vi "DIO0 trigger.vi"(7 "Pulse ticks":u32=2, 8 "error in":errorcluster) -> (0 "error out":errorcluster)   [LabVIEW 2024]
uses:
  <vilib>/rvi/eio/common/nirviEmuTemplateMethod_errors.vi
  <vilib>/eio/EIONode/EIONode.xnode
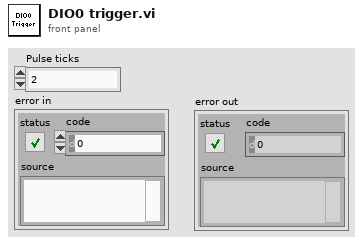
[diagram p1: front panel]
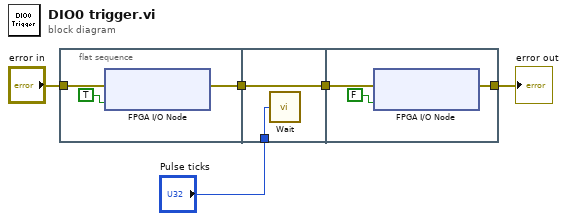
[diagram p0: block diagram]
diagram:
  n1 = flat-sequence {
    tunnel: "error in" -> [w7]
    tunnel: [w6] -> w2
    tunnel: "Pulse ticks" -> [w10]
    tunnel: [w9] -> w3
    tunnel: w2 -> [w9]
    tunnel: w3 -> [w12]
    tunnel: [w11] -> w1
    frame #0 {
      n2 = xnode "FPGA I/O Node"("error in"=w7, "Mod2/DIO0"=TRUE) -> ("error out"=w6:errorcluster)  [unwired: 1 in, 1 out]
    }
    frame #1 {
      n3 = call "Wait"("Count(Ticks)"=w10) -> ()  [unwired: 1 out]
    }
    frame #2 {
      n4 = xnode "FPGA I/O Node"("error in"=w12, "Mod2/DIO0"=FALSE) -> ("error out"=w11:errorcluster)  [unwired: 1 in, 1 out]
    }
  }
  "error out" <- w1
